vi "CPP_ExponentialDecayFit.vi"(2 "SamplingRate":dbl, 3 "DecayData":dbl[](array[numeric])) -> (0 "graphCluster":T1, 1 "decayConstant":dbl)   [LabVIEW 2011]
uses:
  <vilib>/measure/mascope.llb/Transition Measurements 1 chan.vi
  <vilib>/Analysis/NI_AALPro.lvlib
  <vilib>/measure/NI_MAPro.lvlib
panel:
  in  "percent level settings":T2={"method"=enum."auto select", "histogram size"=256, "histogram method"=enum."mode", "reserved"=1.0} {"reserved" format="%0.2f"}
  in  "reference levels":T3={"high ref level"=90.0, "mid ref level"=50.0, "low ref level"=10.0, "ref units"=1} {"ref units" items=["absolute", "percent"]; "high ref level" format="%0.2f"; "low ref level" format="%0.2f"; "mid ref level" format="%0.2f"}
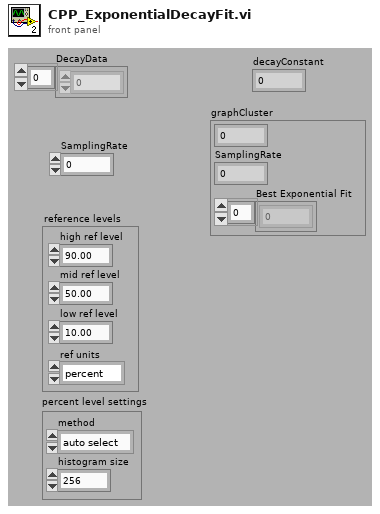
[diagram p1: front panel]
types:
  T1 = cluster{dbl, "SamplingRate":dbl, "Best Exponential Fit":dbl[]}
  T2 = cluster{"method":enum32{"histogram", "peak", "auto select"}, "histogram size":i32, "histogram method":enum16{"mode"}, "reserved":dbl}
  T3 = cluster{"high ref level":dbl, "mid ref level":dbl, "low ref level":dbl, "ref units":u16}
  T4 = cluster{"start time":dbl, "end time":dbl, "ref levels":cluster{"high ref level":dbl, "mid ref level":dbl, "low ref level":dbl, "ref units":u16}}
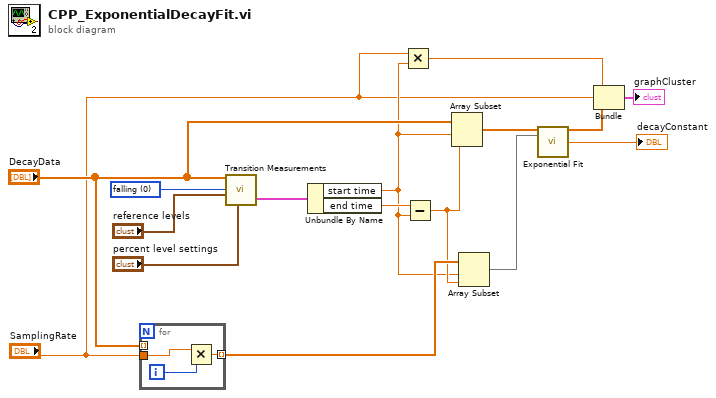
[diagram p0: block diagram]
diagram:
  w15 = u16 0 items=["falling", "rising"] ("polarity (rising)")
  n1 = for {
    tunnel: "DecayData" -> [_] mode=indexing
    tunnel: "SamplingRate" -> [w18]
    tunnel: [w17] -> w9 mode=indexing
    i -> [w19]
    n2 = Multiply(x=w18, y=w19) -> (x*y=w17:dbl)
  }
  n3 = call-poly <vilib>:"Transition Measurements.vi"("percent level settings"="percent level settings", "reference levels"="reference levels", "polarity (rising)"=w15, "signal in"="DecayData") -> ("measurement info"=w13:T4)  [unwired: 2 in, 5 out]
  n4 = Unbundle By Name(w13) -> ("start time"=w5:dbl, "end time"=w12:dbl)
  n5 = Multiply(x="SamplingRate", y=w5) -> (x*y=w4:dbl)
  n6 = Subtract(x=w12, y=w5) -> (x-y=w8:dbl)
  n7 = Array Subset(array="DecayData", index=w5, length=w8) -> (w11:dbl[])
  n8 = Array Subset(array=w9, index=w5, length=w8) -> (w7:dbl[])
  n9 = call <vilib>:"Exponential Fit.vi"("Y"=w11, "X"=w7) -> ("Best Exponential Fit"=w6:dbl[], "damping"=→"decayConstant":dbl)  [unwired: 8 in, 4 out]
  n10 = Bundle(w4, "SamplingRate"="SamplingRate", "Best Exponential Fit"=w6) -> (→"graphCluster":T1)  [unwired: 1 out]
